vi "Ballard XML Generator.XML Version.vi"(10 "version (1.0)":string="1.0", 11 "string in":string) -> (3 "string out":string)   [LabVIEW 2020]
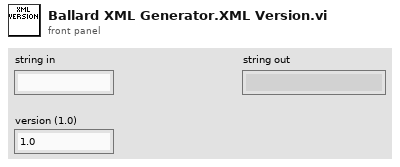
[diagram p1: front panel]
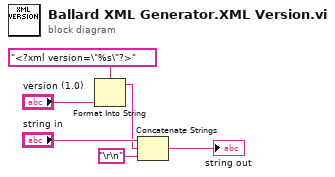
[diagram p0: block diagram]
diagram:
  n1 = Format Into String(format string="<?xml version=\"%s\"?>", "version (1.0)") -> (resulting string=w3:string)  [unwired: 2 in, 1 out]
  n2 = Concatenate Strings("string in", w3, "\r\n") -> (→"string out":string)
